vi "Write Channel Data Offsets.vi"(8 "error in (no error)":errorcluster, 10 "channel data offsets":cluster{"error counts":u32}, 11 "Ballard ARINC-429 Rx Execution Unit in":refnum<class "Rx Execution Unit.lvclass">) -> (0 "error out":errorcluster, 3 "Ballard ARINC-429 Rx Execution Unit out":refnum<class "Rx Execution Unit.lvclass">)   [LabVIEW 2020, in "Ballard ARINC 429 Engine.lvlib" / "Implementation.lvlib" / "Rx Execution Unit.lvclass"]
uses:
  Rx Execution Unit.lvclass
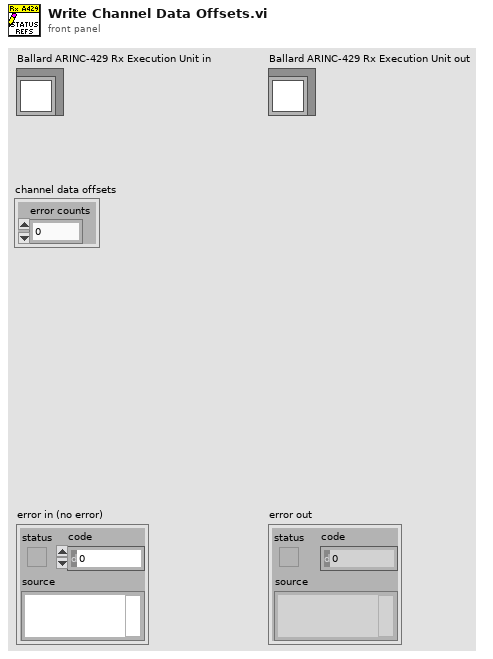
[diagram p1: front panel]
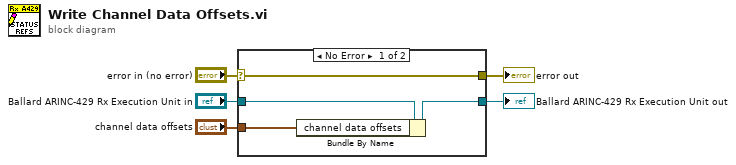
[diagram p0: block diagram]
diagram:
  n1 = case shown="No Error" "error in (no error)" {
    selector: "error in (no error)" -> [w9 w10]
    tunnel: [w9 w10] -> w4
    tunnel: [w7 w11] -> w2
    tunnel: "Ballard ARINC-429 Rx Execution Unit in" -> [w8 w11]
    tunnel: "channel data offsets" -> [w6 _]
    frame No Error {
      n2 = Bundle By Name(cluster=w8, "channel data offsets"=w6) -> (w7:refnum<class "Rx Execution Unit.lvclass">)
    }
    frame Error {
    }
  }
  "error out" <- w4
  "Ballard ARINC-429 Rx Execution Unit out" <- w2
